vi "Load Dark Array Data.vi"(11 "file path (dialog if empty)":path) -> (1 "Freq":dbl[](array[numeric]), 2 "intTime":dbl[](array[numeric]), 3 "Scans":dbl[][](array[numeric]))   [LabVIEW 2013]
uses:
  <vilib>/Utility/file.llb/Read From Spreadsheet File (DBL).vi
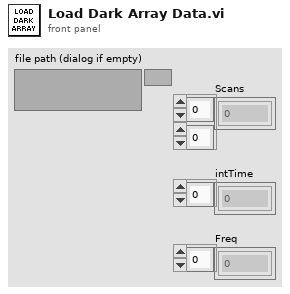
[diagram p1: front panel]
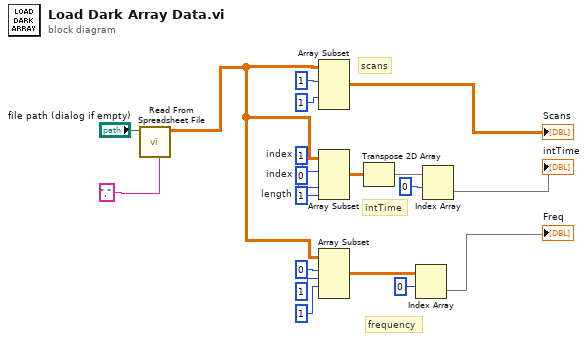
[diagram p0: block diagram]
diagram:
  w5 = 0  # index
  w7 = 1  # length
  w4 = 1  # index
  # "scans"
  # "frequency"
  # "intTime"
  n1 = call-poly <vilib>:"Read From Spreadsheet File.vi"("delimiter (\\t)"="," ("delimiter (\\t)"), "file path (dialog if empty)"="file path (dialog if empty)") -> ("all rows"=w2:dbl[][])  [unwired: 5 in, 4 out]
  n2 = Array Subset(array=w2, index (row)=1 ("length"), index (col)=1 ("length")) -> (→"Scans":dbl[][])  [unwired: 2 in]
  n3 = Array Subset(array=w2, index (row)=w4, index (col)=w5, length (col)=w7) -> (w16:dbl[][])  [unwired: 1 in]
  n4 = Array Subset(array=w2, index (row)=0 ("length"), length (row)=1 ("length"), index (col)=1 ("length")) -> (w15:dbl[][])  [unwired: 1 in]
  n5 = Transpose 2D Array(2D array=w16) -> (transposed array=w17:dbl[][])
  n6 = Index Array(array=w15, index (row)=0) -> (element=→"Freq":dbl[])  [unwired: 1 in]
  n7 = Index Array(array=w17, index (row)=0) -> (element=→"intTime":dbl[])  [unwired: 1 in]
